vi "Process.vi"(8 "error in":errorcluster, 11 "Example Instrument UI":refnum<class "LevyLab Instrument UI.lvclass">) -> (0 "error out":errorcluster, 3 "Example Instrument UI out":refnum<class "LevyLab Instrument UI.lvclass">)   [LabVIEW 2016, in "LevyLab Instrument UI.lvclass"]
doc: "---------------------------------------------------------------\nJKI State Machine Objects™\nhttp://jki.net/state-machine-objects/\nCopyright (C) 2005-2015, JKI <info@jki.net>\nALL RIGHTS RESERVEDJKI State Machine Objects (SMO) 1.0.0.5\nJKI - JKI\nCopyright (c) 2016, JKI"
uses:
  LevyLab Instrument UI.lvclass
  C:/Program Files (x86)/National Instruments/LabVIEW 2016/vi.lib/JKI/JKI SMO/SMO/SMO.lvclass
  C:/Users/patrick/Documents/GitHub/Instrument-Framework/lvsrc/SMOs/Instrument UI/Instrument UI.lvclass
  C:/Program Files (x86)/National Instruments/LabVIEW 2016/vi.lib/JKI/JKI SMO/SMO.UI/SMO.UI.lvclass
  <vilib>/JKI/JKI SMO/SMO/Typedefs/Parent Call--Enum.ctl
  LevyLab Instrument/Typedefs/LevyLab Instrument.getAll--Cluster.ctl
  LevyLab Instrument/LevyLab Instrument.lvclass
  C:/Users/patrick/Documents/GitHub/Instrument-Framework/lvsrc/SMOs/Instrument/Instrument.lvclass
  SMOs/Instrument UI/Instrument UI.lvclass/Instrument UI.ctl
  SMOs/Instrument/Instrument.lvclass
  SMOs/Instrument UI/Instrument UI.lvclass
  <vilib>/JKI/JKI SMO/SMO/SMO.lvclass
  <vilib>/JKI/JKI SMO/SMO.UI/SMO.UI.lvclass
panel:
  out "Numeric":u32
  out "Instrument Response":dbl
  in  "Set Parameter":bool
  in  "Parameter":dbl
  in  "STOP":bool
  out "SMO string":string
  out "SMO Boolean":bool
  out "Logger SMO":dbl
  out "Levy 1":dbl
  # "#todo\nmake UI here. maybe include a nice picture of the hardware?"
  # "#todo\nadd buttons to do stuff (e.g., change a setting)\nButtons should trigger an event"
  # "#todo\nresize this box if you want your UI to be different size"
  # "SMO UI Template"
  # "For instructions on how to use the JKI State Machine Objects, examples and video tutorials, visit:\nhttp://jki.net/state-machine-objects/\n\nJKI State Machine Objects™\nhttp://jki.net/state-machine-objects/\nCopyright (C) 2005-2015, JKI <info@jki.net>\nALL RIGHTS RESERVED"
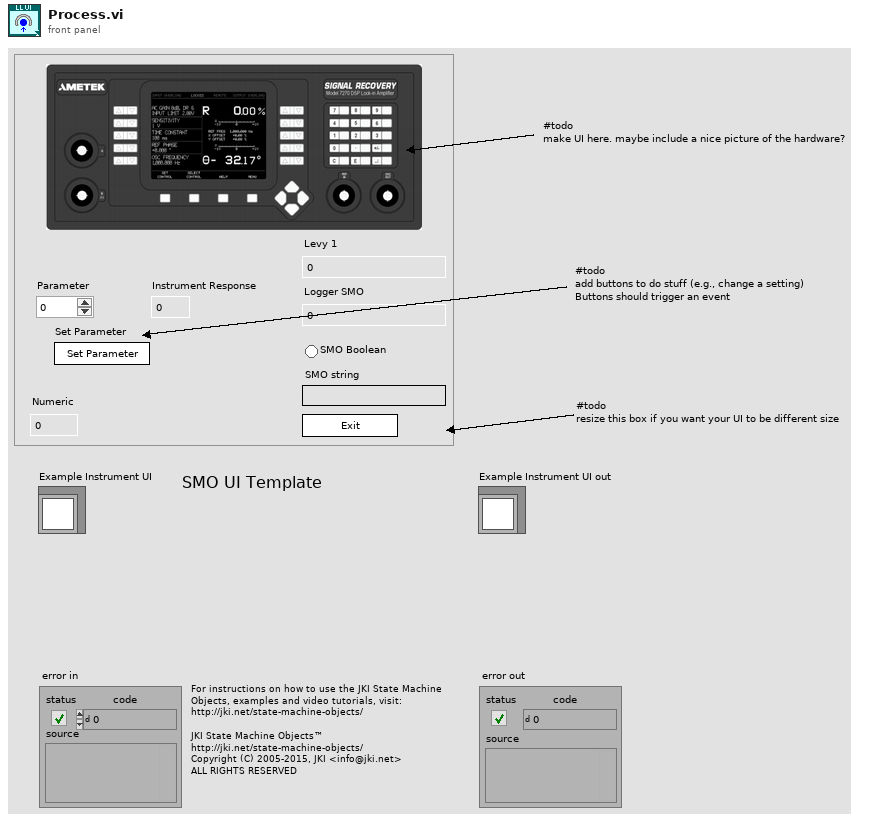
[diagram p1: front panel]
types:
  T1 = typedef "SMO.lvclass/Parent Call--Enum.ctl" = enum16{"Allows parent to run", "Does not request parent to run"}
  T2 = enum32{"invalid app kind", "Development System", "Run Time System", "Student Edition", "Embedded LabVIEW", "Evaluation", "Custom"}
  T3 = enum32{"Invalid", "Standard", "Closed", "Hidden", "Minimized", "Maximized"}
  T4 = typedef "LevyLab Instrument.lvclass/LevyLab Instrument.getAll--Cluster.ctl" = cluster{"Levy 1":dbl, "Logger SMO":dbl, "SMO Boolean":bool, "SMO String":string}
  T5 = cluster{"Core":cluster{"Current VI Reference":refnum<vi>, "Close Panel on Exit?":bool, "error":errorcluster}, "Instrument UI out":refnum<class "LevyLab Instrument UI.lvclass">, "Instrument":refnum<class "LevyLab Instrument.lvclass">, "getAll":T4, "Parameter":dbl}
  T6 = cluster{"Current VI Reference":refnum<vi>, "Close Panel on Exit?":bool, "error":errorcluster}
  T7 = typedef "SMO.lvclass/Protected Events.ctl" = cluster{"StopProcesses":refnum<user-event>, "AbortProcesses":refnum<user-event>, "Config Changed":refnum<user-event>, "Dependency":refnum<user-event>}
  T8 = typedef "Instrument.lvclass/PublicEvents--Cluster.ctl" = cluster{"MessageFromProcess":refnum<user-event>}
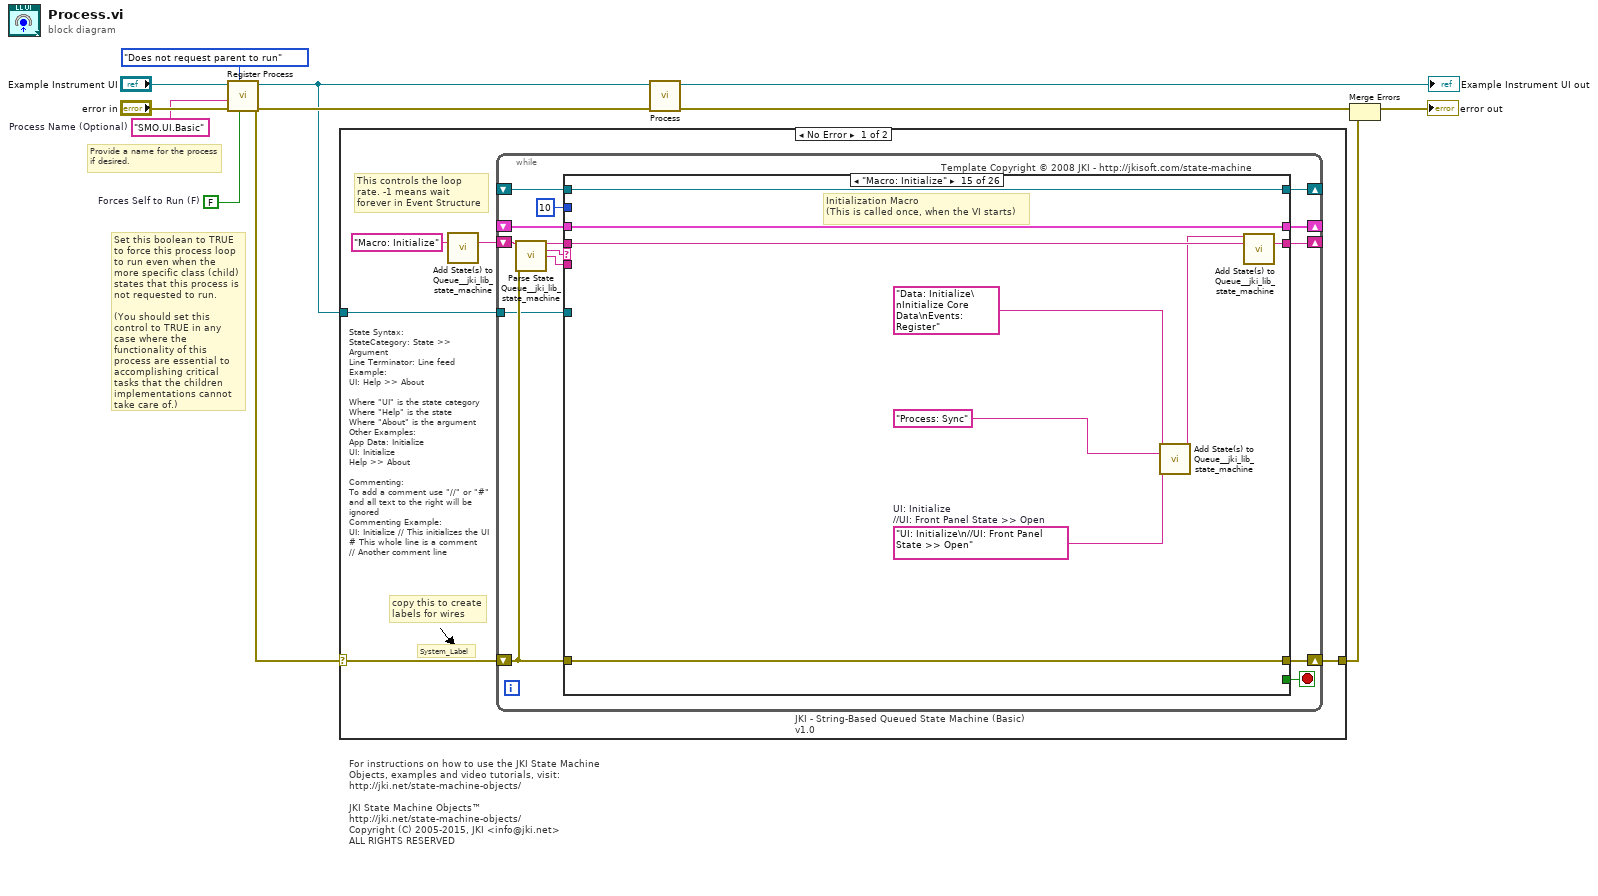
[diagram p0: block diagram]
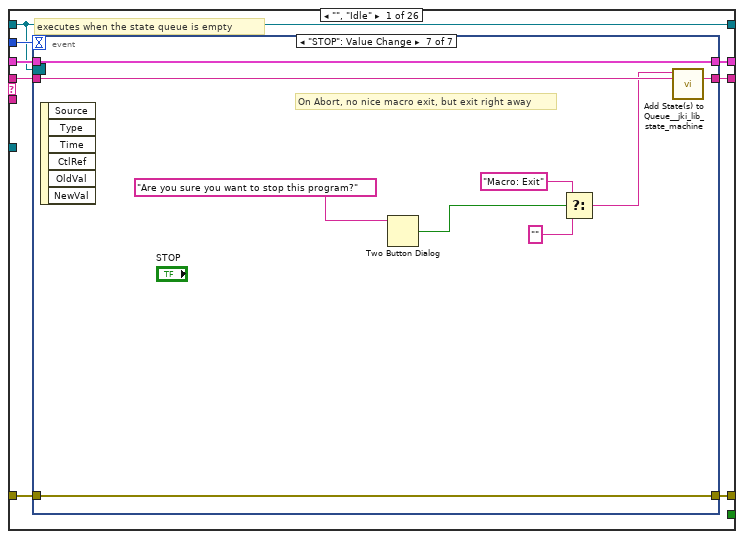
[diagram p2: hidden frame]
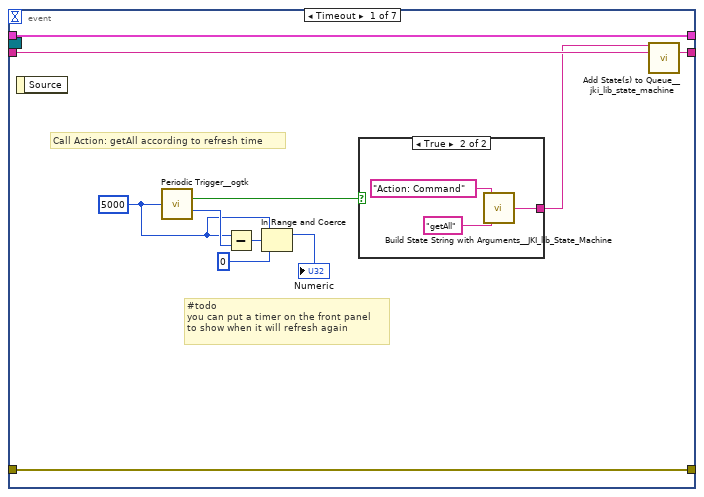
[diagram p3: hidden frame]
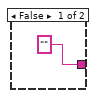
[diagram p4: hidden frame]
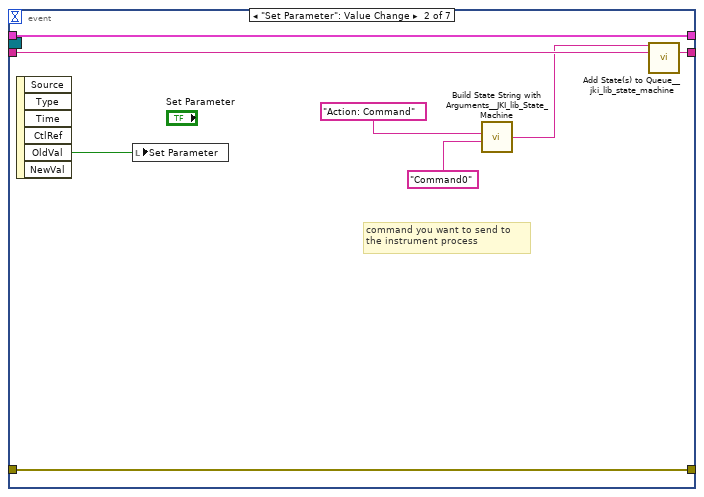
[diagram p5: hidden frame]
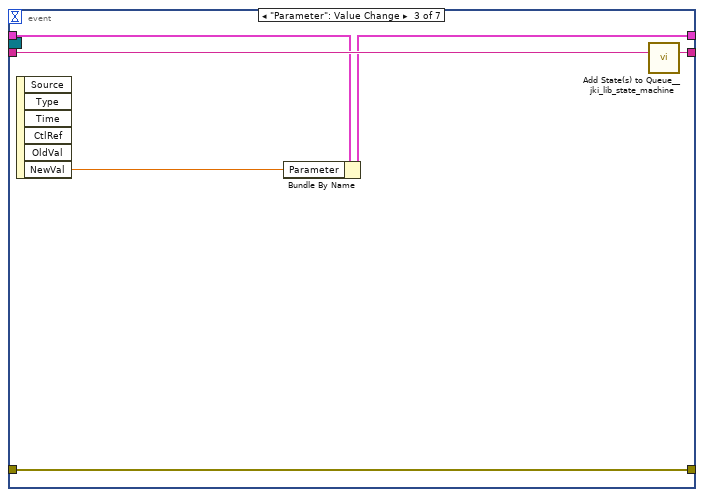
[diagram p6: hidden frame]
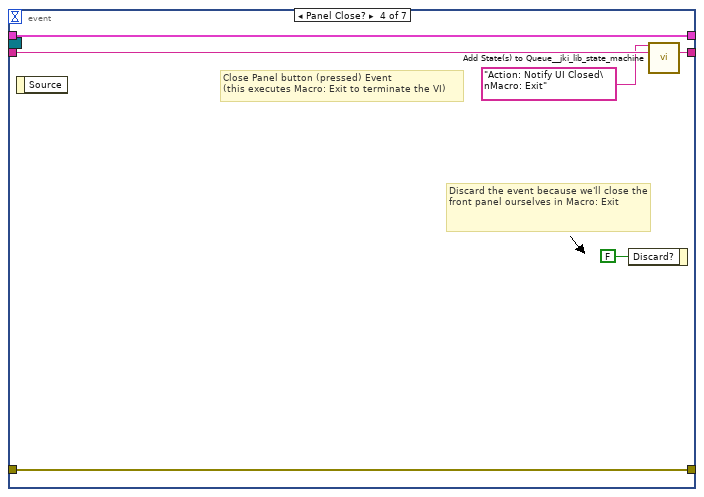
[diagram p7: hidden frame]
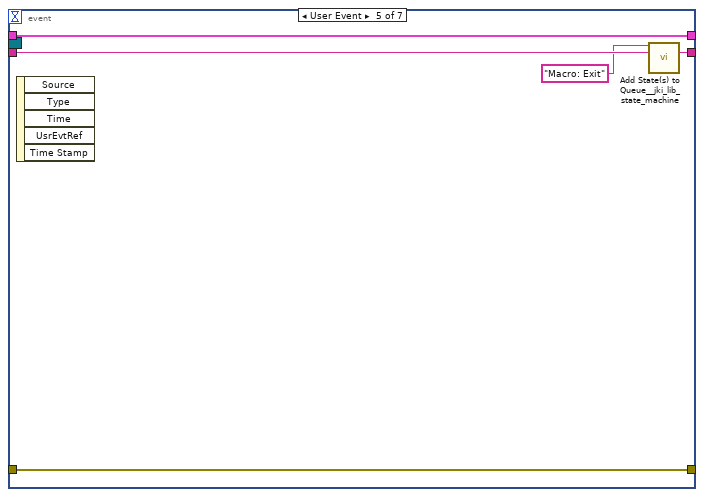
[diagram p8: hidden frame]
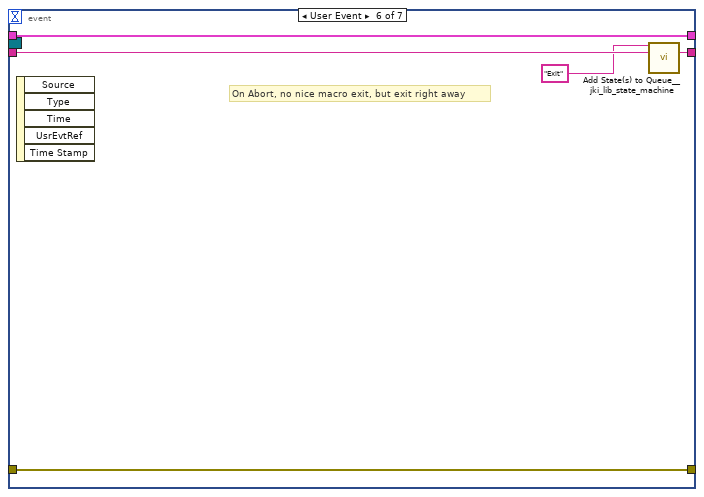
[diagram p9: hidden frame]
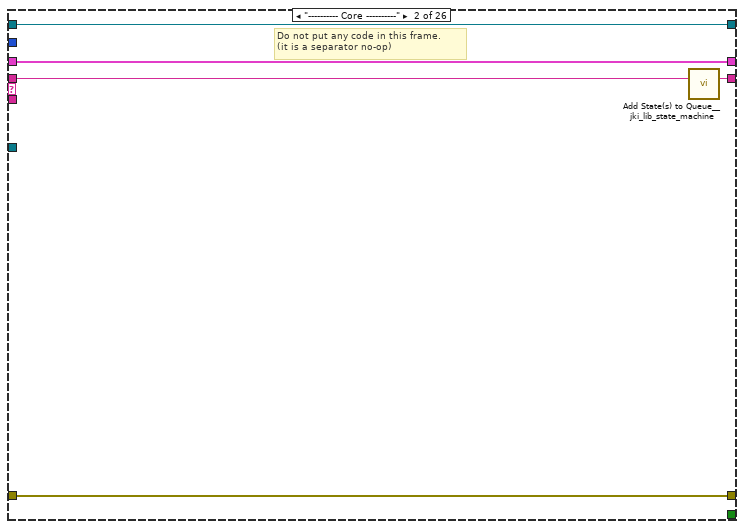
[diagram p10: hidden frame]
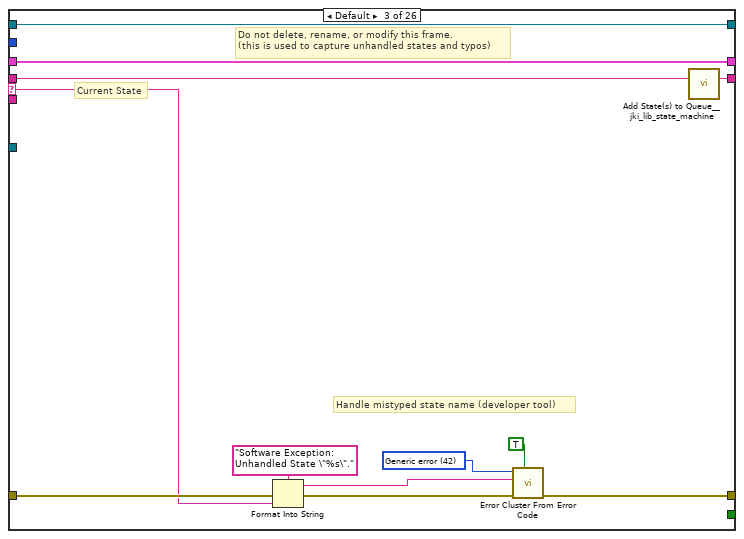
[diagram p11: hidden frame]
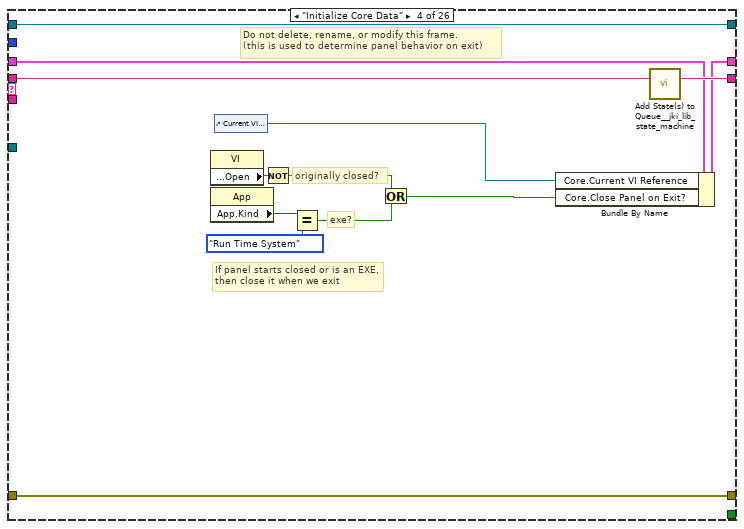
[diagram p12: hidden frame]
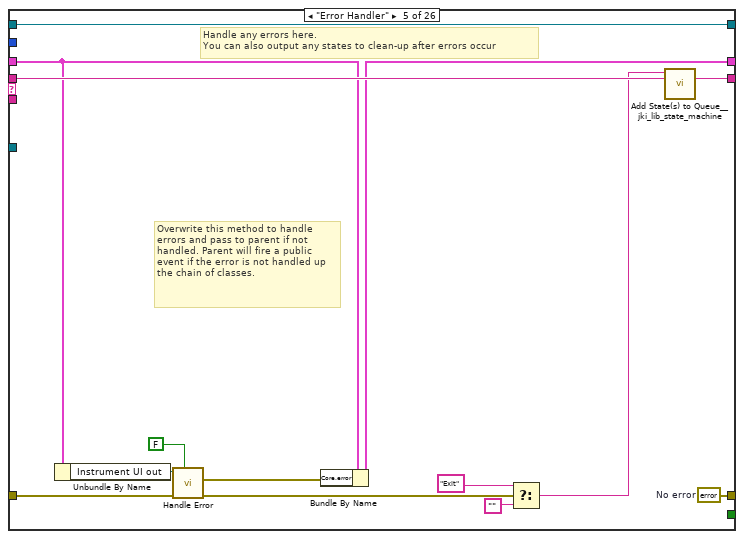
[diagram p13: hidden frame]
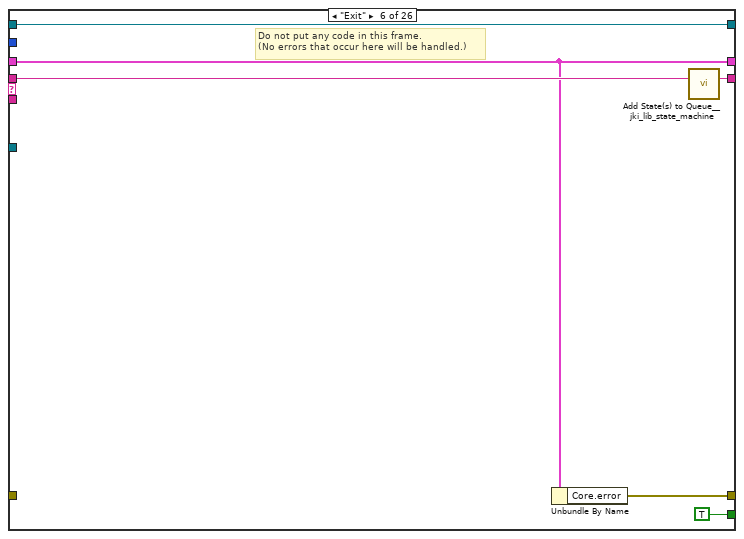
[diagram p14: hidden frame]
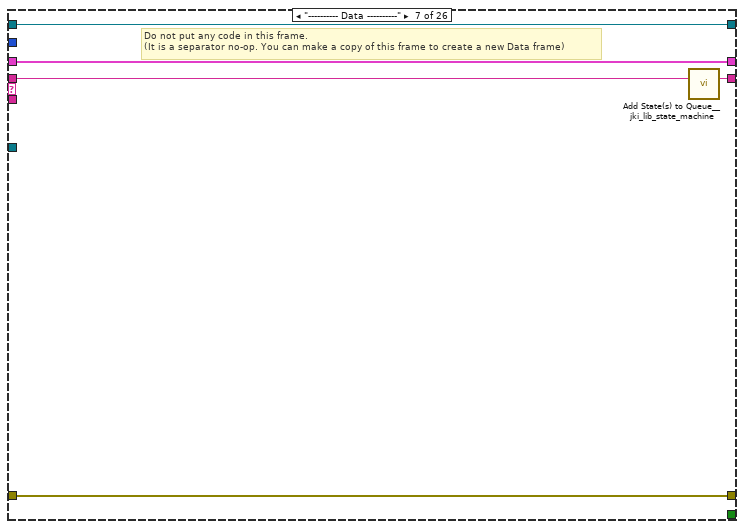
[diagram p15: hidden frame]
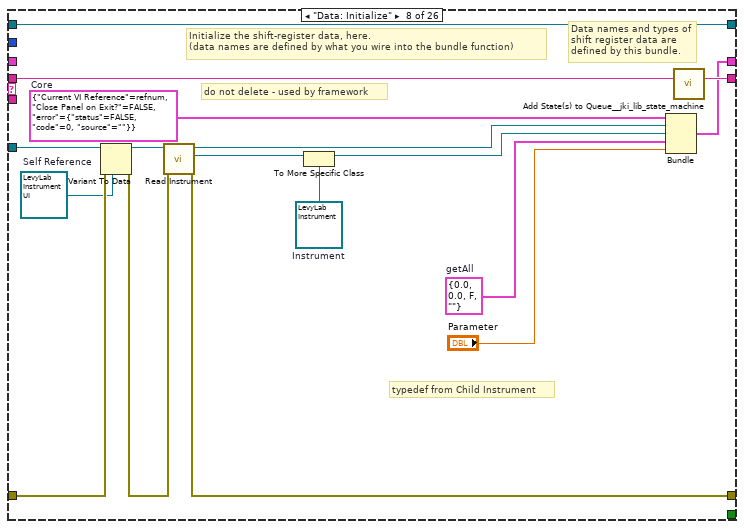
[diagram p16: hidden frame]
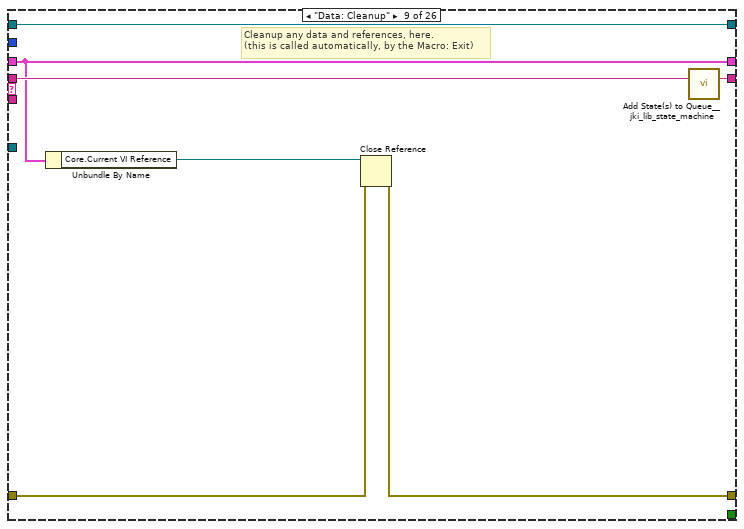
[diagram p17: hidden frame]
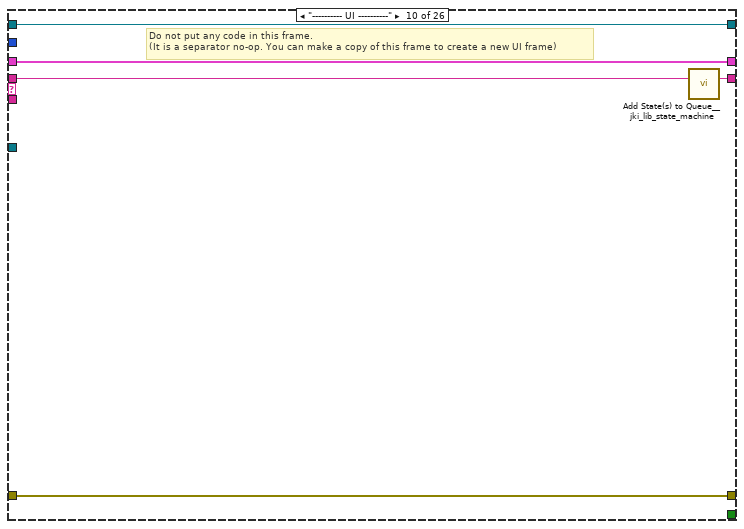
[diagram p18: hidden frame]
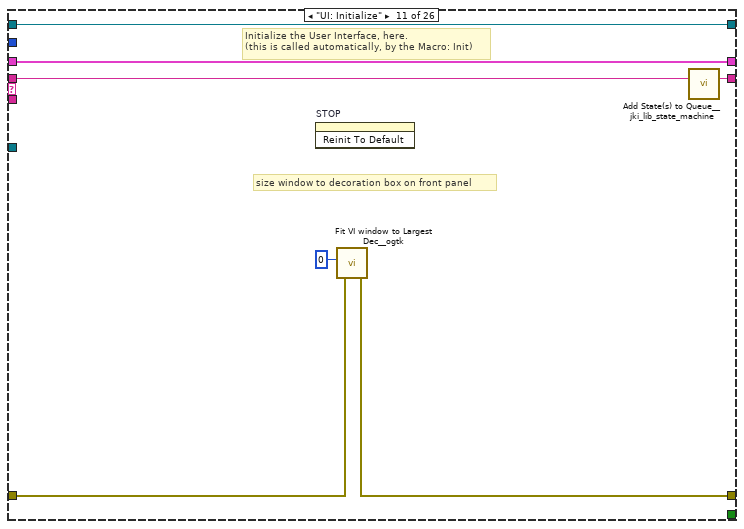
[diagram p19: hidden frame]
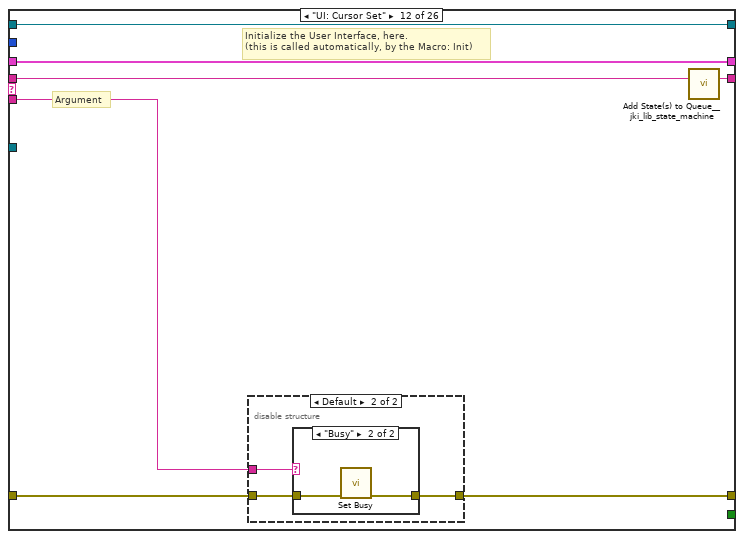
[diagram p20: hidden frame]
diagram:
  w2 = FALSE  # Forces Self to Run (F)
  w1 = "SMO.UI.Basic"  # Process Name (Optional)
  # "Provide a name for the process\nif desired."
  # "Set this boolean to TRUE to force this process loop to run even when the more specific class (child) states that this process is not requested to run.\n\n(You should set this control to TRUE in any case where the functionality of this process are essential to accomplishing critical tasks that the children implementations cannot take care of.)"
  # "For instructions on how to use the JKI State Machine Objects, examples and video tutorials, visit:\nhttp://jki.net/state-machine-objects/\n\nJKI State Machine Objects™\nhttp://jki.net/state-machine-objects/\nCopyright (C) 2005-2015, JKI <info@jki.net>\nALL RIGHTS RESERVED"
  n1 = call <vilib>:"Register Process.vi"("Forces Self to Run (F)"=w2, "Parent Call"=Parent_Call--Enum."Does not request parent to run", "error in (no error)"="error in", "Process Name (optional)"=w1, "SMO"="Example Instrument UI") -> ("error out"=w8:errorcluster, "SMO out"=w7:refnum<class "LevyLab Instrument UI.lvclass">)  [unwired: 5 in]
  n2 = case shown="No Error" w8 {
    selector: w8 -> [w13 w364]
    tunnel: w7 -> [w14 _]
    tunnel: [w12 w364] -> w4
    frame No Error {
      # "State Syntax:\nStateCategory: State >> Argument\nLine Terminator: Line feed\nExample:\nUI: Help >> About\n\nWhere \"UI\" is the state category\nWhere \"Help\" is the state\nWhere \"About\" is the argument\nOther Examples:\nApp Data: Initialize\nUI: Initialize\nHelp >> About\n\nCommenting:\nTo add a comment use \"//\" or \"#\" and all text to the right will be ignored\nCommenting Example:\nUI: Initialize // This initializes the UI\n# This whole line is a comment\n// Another comment line"
      # "copy this to create labels for wires"
      # "This controls the loop rate. -1 means wait forever in Event Structure"
      # "System_Label"
      n3 = call <vilib>:"Add State(s) to Queue__jki_lib_state_machine.vi"("State(s) in (\"\")"="Macro: Initialize") -> ("States Out"=w16:string)  [unwired: 14 in]
      n4 = while "JKI - String-Based Queued State Machine (Basic) v1.0" {
        shift-right: [w23] -> _
        shift-left: _ -> [w22]
        shift-right: [w26] -> w12
        shift-left: w13 -> [w20]
        shift-right: [w25] -> _
        shift-left: w16 -> [w27]
        tunnel: w14 -> [w19]
        shift-right: [w18] -> _
        shift-left: _ -> [w17]
        stop <- w24 stop-if-true
        # "Template Copyright © 2008 JKI - http://jkisoft.com/state-machine"
        n5 = call <vilib>:"Parse State Queue__jki_lib_state_machine.vi"("State Queue"=w27, "Error In (no error)"=w20) -> ("Remaining States"=w29:string, "Current State"=w30:string, "Arguments"=w28:string)  [unwired: 11 in]
        n6 = case shown="\"Macro: Initialize\"" w30 {
          selector: w30 -> [_ _ w99 _ _ _ _ _ _ _ _ _ _ _ _ _ _ _ _ _ _ _ _ _ _ _]
          tunnel: w29 -> [w38 w97 w103 w122 w136 w142 w147 w164 w171 w176 w183 w190 w206 w238 w247 w261 w266 w277 w284 w289 w302 w308 w315 w322 w332 w343]
          tunnel: w28 -> [_ _ _ _ _ _ _ _ _ _ _ w184 w200 _ _ _ _ _ _ _ _ _ _ _ _ w337]
          tunnel: w22 -> [w36 w94 w101 w113 w125 w138 w144 _ w166 w173 w181 w188 w202 w235 w243 w248 w263 w274 w279 w286 w300 w306 w311 w318 w329 w334]
          tunnel: [w35 w95 w105 w119 w127 w137 w145 w151 w167 w174 w178 w185 w203 w236 w245 w259 w264 w268 w280 w287 w295 w303 w312 w316 w323 w340] -> w26
          tunnel: w20 -> [w34 w95 w104 w119 w132 _ w145 w161 w168 w174 w179 w186 w204 w236 w245 w259 w264 w269 w281 w287 w297 w304 w312 w317 w323 w335]
          tunnel: [w37 w96 w102 w121 w135 w141 w146 w163 w170 w175 w182 w189 w205 w237 w246 w260 w265 w276 w283 w288 w301 w307 w314 w321 w331 w342] -> w25
          tunnel: [_ _ _ _ _ TRUE _ _ _ _ _ _ _ _ _ _ _ _ _ _ _ _ _ _ _ _] -> w24
          tunnel: [w33 w94 w101 w120 w124 w138 w144 w162 w166 w173 w181 w188 w202 w235 w243 w248 w263 w274 w279 w286 w300 w306 w310 w318 w329 w333] -> w23
          tunnel: 10 ("Timeout") -> [w32 _ _ _ _ _ _ _ _ _ _ _ _ _ _ _ _ _ _ _ _ _ _ _ _ _]
          tunnel: w19 -> [_ _ _ _ _ _ _ w159 _ _ _ _ _ _ _ _ _ _ _ _ _ _ _ _ _ _]
          tunnel: [w31 w93 w98 w110 w134 w139 w143 w158 w165 w172 w180 w187 w199 w234 w244 w253 w262 w275 w282 w285 w299 w305 w313 w320 w330 w341] -> w18
          tunnel: w17 -> [w31 w93 w98 w110 w134 w139 w143 w158 w165 w172 w180 w187 w199 w234 w244 w253 w262 w275 w282 w285 _ w305 w313 w320 w330 w341]
          frame "", "Idle" {
            # "executes when the state queue is empty"
            n7 = event shown="[6] \"STOP\": Value Change" {
              selector: w31 -> [_ _ _ _ _ _ _]
              dyn-events: _ -> [_ _ _ _ _ _ _]
              timeout: w32 -> [_ _ _ _ _ _ _]
              tunnel: w38 -> [w49 w61 w67 w73 w78 w83 w92]
              tunnel: [w48 w60 w66 w72 w77 w82 w91] -> w37
              tunnel: w36 -> [w46 w58 w63 w69 w75 w80 w89]
              tunnel: [w47 w59 w65 w68 w76 w81 w90] -> w35
              tunnel: w34 -> [w47 w59 w65 w68 w76 w81 w90]
              tunnel: [w46 w58 w62 w69 w75 w80 w89] -> w33
              event Timeout {
                w40 = u32 5000 ("time (ms)")
                # "#todo\nyou can put a timer on the front panel\nto show when it will refresh again"
                # "Call Action: getAll according to refresh time"
                n8 = event-data() -> ()  [unwired: 1 in, 1 out]
                n9 = call <userlib>:"Periodic Trigger__ogtk.vi"("time (ms)"=w40) -> ("Triggered"=w44:bool, "timer value"=w43:u32)  [unwired: 12 in, 1 out]
                n10 = Subtract(x=w40, y=w43) -> (x-y=w42:u32)
                n11 = In Range and Coerce(upper limit=w40, x=w42, lower limit=u32 0) -> (coerced(x)=→"Numeric":u32)  [unwired: 1 out]
                n12 = case shown="True" w44 {
                  tunnel: ["" ("State(s) in Front (\"\")") w51] -> w45
                  frame False {
                  }
                  frame True {
                    n13 = call <vilib>:"Build State String with Arguments__JKI_lib_State_Machine.vi"("Arguments (\"\")"="getAll" ("State(s) in Front (\"\")"), "State"="Action: Command" ("State(s) in Front (\"\")")) -> ("State with Arguments"=w51:string)  [unwired: 4 in]
                  }
                }
                n14 = call <vilib>:"Add State(s) to Queue__jki_lib_state_machine.vi"("State(s) in Front (\"\")"=w45, "State(s) in (\"\")"=w49) -> ("States Out"=w48:string)  [unwired: 13 in]
              }
              event "Set Parameter": Value Change {
                # "command you want to send to\nthe instrument process"
                n15 = event-data() -> ("OldVal"=w57:bool)  [unwired: 1 in, 5 out]
                n16 = local write "Set Parameter"(w57) -> ()
                n17 = call <vilib>:"Build State String with Arguments__JKI_lib_State_Machine.vi"("Arguments (\"\")"="Command0" ("State(s) in Front (\"\")"), "State"="Action: Command" ("State(s) in Front (\"\")")) -> ("State with Arguments"=w54:string)  [unwired: 4 in]
                n18 = call <vilib>:"Add State(s) to Queue__jki_lib_state_machine.vi"("State(s) in Front (\"\")"=w54, "State(s) in (\"\")"=w61) -> ("States Out"=w60:string)  [unwired: 13 in]
              }
              event "Parameter": Value Change {
                n19 = event-data() -> ("NewVal"=w64:dbl)  [unwired: 1 in, 5 out]
                n20 = Bundle By Name(cluster=w63, "Parameter"=w64) -> (w62:T5)
                n21 = call <vilib>:"Add State(s) to Queue__jki_lib_state_machine.vi"("State(s) in (\"\")"=w67) -> ("States Out"=w66:string)  [unwired: 14 in]
              }
              event Panel Close? {
                # "Discard the event because we'll close the front panel ourselves in Macro: Exit"
                # "Close Panel button (pressed) Event\n(this executes Macro: Exit to terminate the VI)"
                n22 = event-data() -> ()  [unwired: 1 in, 1 out]
                n23 = event-data("Discard?"=FALSE) -> ()  [unwired: 1 in, 1 out]
                n24 = call <vilib>:"Add State(s) to Queue__jki_lib_state_machine.vi"("State(s) in Front (\"\")"="Action: Notify UI Closed\nMacro: Exit", "State(s) in (\"\")"=w73) -> ("States Out"=w72:string)  [unwired: 13 in]
              }
              event User Event {
                n25 = event-data() -> ()  [unwired: 1 in, 5 out]
                n26 = call <vilib>:"Add State(s) to Queue__jki_lib_state_machine.vi"("State(s) in Front (\"\")"="Macro: Exit", "State(s) in (\"\")"=w78) -> ("States Out"=w77:string)  [unwired: 13 in]
              }
              event User Event {
                # "On Abort, no nice macro exit, but exit right away"
                n27 = event-data() -> ()  [unwired: 1 in, 5 out]
                n28 = call <vilib>:"Add State(s) to Queue__jki_lib_state_machine.vi"("State(s) in Front (\"\")"="Exit", "State(s) in (\"\")"=w83) -> ("States Out"=w82:string)  [unwired: 13 in]
              }
              event "STOP": Value Change {
                # "On Abort, no nice macro exit, but exit right away"
                n29 = event-data() -> ()  [unwired: 1 in, 6 out]
                n30 = Two Button Dialog(message="Are you sure you want to stop this program?") -> (T button?=w88:bool)  [unwired: 2 in]
                n31 = Select(t="Macro: Exit", s=w88, f="") -> (s? t:f=w84:string)
                n32 = call <vilib>:"Add State(s) to Queue__jki_lib_state_machine.vi"("State(s) in Front (\"\")"=w84, "State(s) in (\"\")"=w92) -> ("States Out"=w91:string)  [unwired: 13 in]
              }
            }
          }
          frame "---------- Core ----------" {
            # "Do not put any code in this frame.\n(it is a separator no-op)"
            n33 = call <vilib>:"Add State(s) to Queue__jki_lib_state_machine.vi"("State(s) in (\"\")"=w97) -> ("States Out"=w96:string)  [unwired: 14 in]
          }
          frame Default {
            w108 = 42 items=["No error", "Argument error", "Memory is full", "Out of zone", "End of file", "File already open", "Generic file I/O error", "File not found", "File permission error", "Disk is full", "Duplicate path", "Too many files open", "System feature not enabled", "Resource file not found", "Cannot add resource", "Resource not found", "Image not found", "Image memory error", "Pen does not exist", "Config type invalid", "Config token not found", "Config parse error", "Config memory error", "Bad external code format", "Bad external code offset", "External code not present", "Null window", "Destroy window error", "Null menu", "Print aborted", "Bad print record", "Print driver error", "Windows error during printing", "Memory error during printing", "Print dialog error", "Generic print error", "Invalid device refnum", "Device not found", "Device parameter error", "Device unit error", "Cannot open device", "Device call aborted", "Generic error", "Cancelled by user", "Object ID too low", "Object ID too high", "Object not in heap", "Unknown heap", "Unknown object (invalid DefProc)", "Unknown object (DefProc not in table)", "Message out of range", "Invalid (null) method", "Unknown message", "Manager call not supported", "Bad address", "Network operation in progress", "Network operation timed out", "Connection is busy", "Network attribute not supported", "Network error", "Address in use", "System out of memory", "Connection aborted", "Connection refused", "Not connected", "Already connected", "Connection closed", "Initialization error (interapplication manager)", "Bad occurrence", "Wait on unbound occurrence handler", "Occurrence queue overflow", "Datalog type conflict", "Unused", "Unrecognized type (interapplication manager)", "Memory corrupt", "Failed to make temporary DLL", "Old CIN version", "Drag socket not found", "Failed to load drop-object", "Failed to register OLE object", "Failed to release OLE object", "Format specifier type mismatch", "Unknown format specifier", "Too few format specifiers", "Too many format specifiers", "Scan failed", "Newer CIN version", "Error converting to variant", "Runtime menu error", "Password tampered", "Variant attribute not found", "Incompatible variant data type", "Event data is not available", "Event Store is not present", "Occurrence is not found", "Event Queue is not created", "Event info is not available", "Refnum passed is NULL", "Error retrieving Class GUID", "Error retrieving CoClass GUID", "Error retrieving TypeLib GUID.", "Bad built application magic bytes.", "Specific driver is different from the specific driver associated with the Logical Name.", "There is no session opened to the class driver.", "Max Error", "MAX - Error with config objects", "MAX - Error loading configuration", "MAX - Group not supported"]
            # "Current State"
            # "Do not delete, rename, or modify this frame.\n(this is used to capture unhandled states and typos)"
            # "Handle mistyped state name (developer tool)"
            n34 = Format Into String(format string="Software Exception: Unhandled State \"%s\"." ("message"), error in=w104, w99) -> (resulting string=w107:string, error out=w106:errorcluster)  [unwired: 1 in]
            n35 = call <vilib>:"Error Cluster From Error Code.vi"("show call chain? (False)"=TRUE, "error in (no error)"=w106, "error message (\"\")"=w107, "error code (0)"=w108) -> ("error out"=w105:errorcluster)  [unwired: 5 in]
            n36 = call <vilib>:"Add State(s) to Queue__jki_lib_state_machine.vi"("State(s) in (\"\")"=w103) -> ("States Out"=w102:string)  [unwired: 14 in]
          }
          frame "Initialize Core Data" {
            # "Do not delete, rename, or modify this frame.\n(this is used to determine panel behavior on exit)"
            # "originally closed?"
            # "exe?"
            # "If panel starts closed or is an EXE, then close it when we exit"
            n37 = property class="VI"() -> ("Front Panel.Open"=w118:bool)  [unwired: 2 in, 2 out]
            n38 = property class="App"() -> ("App.Kind"=w117:T2)  [unwired: 2 in, 2 out]
            n39 = control-ref of="Current VI Reference"() -> (w111:refnum<vi>)
            n40 = Not(x=w118) -> (.not. x?=w115:bool)
            n41 = Equal?(x=w117, y=T2."Run Time System" ("Application:Kind")) -> (x = y?=w114:bool)
            n42 = Or(x=w115, y=w114) -> (x .or. y?=w112:bool)
            n43 = Bundle By Name(cluster=w113, "Core.Current VI Reference"=w111, "Core.Close Panel on Exit?"=w112) -> (w120:T5)
            n44 = call <vilib>:"Add State(s) to Queue__jki_lib_state_machine.vi"("State(s) in (\"\")"=w122) -> ("States Out"=w121:string)  [unwired: 14 in]
          }
          frame "Error Handler" {
            w127 = errorcluster {"status"=FALSE, "code"=0, "source"=""}  # No error
            # "Overwrite this method to handle errors and pass to parent if not handled. Parent will fire a public event if the error is not handled up the chain of classes."
            # "Handle any errors here.\nYou can also output any states to clean-up after errors occur"
            n45 = Unbundle By Name(w125) -> ("Instrument UI out"=w133:refnum<class "LevyLab Instrument UI.lvclass">)
            n46 = call-dynamic "Handle Error.vi"("Stop on Unhandled Error (T)"=FALSE, "error in"=w132, "Instrument UI"=w133) -> ("handling error"=w128:errorcluster, "Unhandled error"=w126:errorcluster)  [unwired: 6 in, 1 out]
            n47 = Bundle By Name(cluster=w125, "Core.error"=w126) -> (w124:T5)
            n48 = Select(t="Exit", s=w128, f="") -> (s? t:f=w129:string)
            n49 = call <vilib>:"Add State(s) to Queue__jki_lib_state_machine.vi"("State(s) in Front (\"\")"=w129, "State(s) in (\"\")"=w136) -> ("States Out"=w135:string)  [unwired: 13 in]
          }
          frame "Exit" {
            # "Do not put any code in this frame.\n(No errors that occur here will be handled.)"
            n50 = Unbundle By Name(w138) -> ("Core.error"=w137:errorcluster)
            n51 = call <vilib>:"Add State(s) to Queue__jki_lib_state_machine.vi"("State(s) in (\"\")"=w142) -> ("States Out"=w141:string)  [unwired: 14 in]
          }
          frame "---------- Data ----------" {
            # "Do not put any code in this frame.\n(It is a separator no-op. You can make a copy of this frame to create a new Data frame)"
            n52 = call <vilib>:"Add State(s) to Queue__jki_lib_state_machine.vi"("State(s) in (\"\")"=w147) -> ("States Out"=w146:string)  [unwired: 14 in]
          }
          frame "Data: Initialize" {
            w154 = refnum<class "LevyLab Instrument.lvclass"> refnum  # Instrument
            w155 = T4 {"Levy 1"=0.0, "Logger SMO"=0.0, "SMO Boolean"=FALSE, "SMO String"=""}  # getAll
            w157 = T6 {"Current VI Reference"=refnum, "Close Panel on Exit?"=FALSE, "error"={"status"=FALSE, "code"=0, "source"=""}}  # Core
            w160 = refnum<class "LevyLab Instrument UI.lvclass"> refnum  # Self Reference
            # "typedef from Child Instrument"
            # "do not delete - used by framework"
            # "Data names and types of shift register data are defined by this bundle."
            # "Initialize the shift-register data, here.\n(data names are defined by what you wire into the bundle function)"
            n53 = Variant To Data(error in=w161, type=w160, Variant=w159) -> (data=w149:refnum<class "LevyLab Instrument UI.lvclass">, error out=w152:errorcluster)
            n54 = call "Read Instrument.vi"("error in (no error)"=w152, "Instrument UI in"=w149) -> ("error out"=w151:errorcluster, "Instrument.lvclass"=w150:refnum<class "Instrument.lvclass">, "Instrument UI out"=w148:refnum<class "LevyLab Instrument UI.lvclass">)  [unwired: 7 in]
            n55 = To More Specific Class(target class=w154, reference=w150) -> (specific class reference=w153:refnum<class "LevyLab Instrument.lvclass">)  [unwired: 1 in, 1 out]
            n56 = Bundle("Core"=w157, "Instrument UI out"=w148, "Instrument"=w153, "getAll"=w155, "Parameter"="Parameter") -> (w162:T5)  [unwired: 1 in]
            n57 = call <vilib>:"Add State(s) to Queue__jki_lib_state_machine.vi"("State(s) in (\"\")"=w164) -> ("States Out"=w163:string)  [unwired: 14 in]
          }
          frame "Data: Cleanup" {
            # "Cleanup any data and references, here.\n(this is called automatically, by the Macro: Exit)"
            n58 = Unbundle By Name(w166) -> ("Core.Current VI Reference"=w169:refnum<vi>)
            n59 = Close Reference(reference=w169, error in (no error)=w168) -> (error out=w167:errorcluster)
            n60 = call <vilib>:"Add State(s) to Queue__jki_lib_state_machine.vi"("State(s) in (\"\")"=w171) -> ("States Out"=w170:string)  [unwired: 14 in]
          }
          frame "---------- UI ----------" {
            # "Do not put any code in this frame.\n(It is a separator no-op. You can make a copy of this frame to create a new UI frame)"
            n61 = call <vilib>:"Add State(s) to Queue__jki_lib_state_machine.vi"("State(s) in (\"\")"=w176) -> ("States Out"=w175:string)  [unwired: 14 in]
          }
          frame "UI: Initialize" {
            # "size window to decoration box on front panel"
            # "Initialize the User Interface, here.\n(this is called automatically, by the Macro: Init)"
            n62 = invoke on="STOP" class="Bool (strict)" method="Reinit To Default"() -> ()  [unwired: 3 in, 3 out]
            n63 = call <userlib>:"Fit VI window to Largest Dec__ogtk.vi"("error in (no error)"=w179, "border spacing (2 px)"=0) -> ("error out"=w178:errorcluster)  [unwired: 4 in, 1 out]
            n64 = call <vilib>:"Add State(s) to Queue__jki_lib_state_machine.vi"("State(s) in (\"\")"=w183) -> ("States Out"=w182:string)  [unwired: 14 in]
          }
          frame "UI: Cursor Set" {
            # "Argument"
            # "Initialize the User Interface, here.\n(this is called automatically, by the Macro: Init)"
            n65 = disable-structure shown="Default" {
              disable-tunnel: w186 -> [w191 w194]
              disable-tunnel: [w191 w193] -> w185
              disable-tunnel: w184 -> [_ w192]
              frame condition #0 {
              }
              frame condition #1 (active) {
                n66 = case shown="\"Busy\"" w192 {
                  tunnel: w194 -> [w196 w198]
                  tunnel: [w195 w197] -> w193
                  frame "Idle", Default {
                    n67 = call <vilib>:"Unset Busy.vi"("error in (no error)"=w196) -> ("error out"=w195:errorcluster)  [unwired: 10 in]
                  }
                  frame "Busy" {
                    n68 = call <vilib>:"Set Busy.vi"("error in (no error)"=w198) -> ("error out"=w197:errorcluster)  [unwired: 9 in, 1 out]
                  }
                }
              }
            }
            n69 = call <vilib>:"Add State(s) to Queue__jki_lib_state_machine.vi"("State(s) in (\"\")"=w190) -> ("States Out"=w189:string)  [unwired: 14 in]
          }
          frame "UI: Front Panel State" {
            # "Argument"
            # "Set Front Panel Open or Closed\n(Usage: \"UI: Front Panel State >> Open|Close\")"
            n70 = Unbundle By Name(w202) -> ("Core.Current VI Reference"=w201:refnum<vi>)
            n71 = disable-structure shown="Default" {
              disable-tunnel: w204 -> [w210 w233]
              disable-tunnel: [w209 w233] -> w203
              disable-tunnel: w201 -> [w208 _]
              disable-tunnel: w200 -> [w207 _]
              frame condition #0 (active) {
                n72 = case shown="\"Close\"" w207 {
                  tunnel: w210 -> [w214 w227]
                  tunnel: [w216 w228] -> w209
                  tunnel: w208 -> [w215 w225]
                  frame "Open", Default {
                    n73 = property class="VI"(reference=w215, error in=w214) -> (reference out=w212:refnum<vi>, error out=w213:errorcluster, "FP.State"=w211:T3)
                    n74 = case shown="\"Closed\"" w211 {
                      tunnel: [w219 w222] -> w216
                      tunnel: w213 -> [w218 w222]
                      tunnel: w212 -> [w217 _]
                      frame "Closed" {
                        n75 = invoke class="VI" method="FP.Open"(reference=w217, error in=w218, "Activate"=TRUE, "State"=T3."Standard") -> (error out=w219:errorcluster)  [unwired: 1 in, 4 out]
                      }
                      frame Default {
                      }
                    }
                  }
                  frame "Close" {
                    n76 = property class="VI"(reference=w225, error in=w227) -> (reference out=w224:refnum<vi>, error out=w226:errorcluster, "FP.State"=w223:T3)
                    n77 = case shown="Default" w223 {
                      tunnel: [w229 w232] -> w228
                      tunnel: w226 -> [w229 w231]
                      tunnel: w224 -> [_ w230]
                      frame "Invalid", "Closed" {
                      }
                      frame Default {
                        n78 = invoke class="VI" method="FP.Close"(reference=w230, error in=w231) -> (error out=w232:errorcluster)  [unwired: 1 in, 2 out]
                      }
                    }
                  }
                }
              }
              frame condition #1 {
              }
            }
            n79 = call <vilib>:"Add State(s) to Queue__jki_lib_state_machine.vi"("State(s) in (\"\")"=w206) -> ("States Out"=w205:string)  [unwired: 14 in]
          }
          frame "---------- Macro ----------" {
            # "Do not put any code in this frame.\n(It is a separator no-op. You can make a copy of this frame to create a new Macro frame)"
            n80 = call <vilib>:"Add State(s) to Queue__jki_lib_state_machine.vi"("State(s) in (\"\")"=w238) -> ("States Out"=w237:string)  [unwired: 14 in]
          }
          frame "Macro: Initialize" {
            w241 = "UI: Initialize\n//UI: Front Panel State >> Open"  # UI: Initialize //UI: Front Panel State >> Open
            # "Initialization Macro\n(This is called once, when the VI starts)"
            n81 = call <vilib>:"Add State(s) to Queue__jki_lib_state_machine.vi"("State(s) in Front (\"\")"="Data: Initialize\nInitialize Core Data\nEvents: Register", "State(s) in (\"\")"="Process: Sync", "State(s) at Back (\"\")"=w241) -> ("States Out"=w240:string)  [unwired: 12 in]
            n82 = call <vilib>:"Add State(s) to Queue__jki_lib_state_machine.vi"("State(s) in Front (\"\")"=w240, "State(s) in (\"\")"=w247) -> ("States Out"=w246:string)  [unwired: 13 in]
          }
          frame "Macro: Exit" {
            # "Exit Macro\n(This is called once, when the VI exits)"
            n83 = Unbundle By Name(w248) -> ("Core.Close Panel on Exit?"=w258:bool)
            n84 = Select(t="UI: Front Panel State >> Close", s=w258, f="") -> (s? t:f=w255:string)
            n85 = call <vilib>:"Add State(s) to Queue__jki_lib_state_machine.vi"("State(s) in Front (\"\")"="Data: Cleanup\nEvents: Unregister\nProcess: Self Terminate", "State(s) in (\"\")"="Process: Sync", "State(s) at Back (\"\")"="Exit") -> ("States Out"=w250:string)  [unwired: 12 in]
            n86 = call <vilib>:"Add State(s) to Queue__jki_lib_state_machine.vi"("State(s) in (\"\")"=w255, "State(s) at Back (\"\")"=w250) -> ("States Out"=w254:string)  [unwired: 13 in]
            n87 = call <vilib>:"Add State(s) to Queue__jki_lib_state_machine.vi"("State(s) in Front (\"\")"=w254, "State(s) in (\"\")"=w261) -> ("States Out"=w260:string)  [unwired: 13 in]
          }
          frame "---------- Process ----------" {
            # "Template Separator\n(You can make a copy of, or modify, this frame)"
            n88 = call <vilib>:"Add State(s) to Queue__jki_lib_state_machine.vi"("State(s) in (\"\")"=w266) -> ("States Out"=w265:string)  [unwired: 14 in]
          }
          frame "Process: Sync" {
            n89 = Unbundle By Name(w274) -> ("Instrument UI out"=w270:refnum<class "LevyLab Instrument UI.lvclass">)
            n90 = call <vilib>:"WaitOnProcessSync.vi"("error in (no error)"=w269, "SMO"=w270) -> ("error out"=w268:errorcluster, "Don't run?"=w273:bool)  [unwired: 7 in, 1 out]
            n91 = Select(t="Data: Cleanup\nEvents: Unregister\nExit", s=w273, f="") -> (s? t:f=w267:string)
            n92 = call <vilib>:"Add State(s) to Queue__jki_lib_state_machine.vi"("State(s) in Front (\"\")"=w267, "State(s) in (\"\")"=w277) -> ("States Out"=w276:string)  [unwired: 13 in]
          }
          frame "Process: Self Terminate" {
            n93 = Unbundle By Name(w279) -> ("Instrument UI out"=w278:refnum<class "LevyLab Instrument UI.lvclass">)
            n94 = call <vilib>:"SelfTerminate.vi"("error in (no error)"=w281, "SMO in"=w278) -> ("error out"=w280:errorcluster)  [unwired: 8 in, 1 out]
            n95 = call <vilib>:"Add State(s) to Queue__jki_lib_state_machine.vi"("State(s) in (\"\")"=w284) -> ("States Out"=w283:string)  [unwired: 14 in]
          }
          frame "---------- Events ----------" {
            # "Template Separator\n(You can make a copy of, or modify, this frame)"
            n96 = call <vilib>:"Add State(s) to Queue__jki_lib_state_machine.vi"("State(s) in (\"\")"=w289) -> ("States Out"=w288:string)  [unwired: 14 in]
          }
          frame "Events: Register" {
            # "Expand to add\nmore events"
            # "Base Class Protected Events"
            n97 = Unbundle By Name(w300) -> ("Instrument UI out"=w290:refnum<class "LevyLab Instrument UI.lvclass">, "Instrument"=w293:refnum<class "LevyLab Instrument.lvclass">)
            n98 = call <vilib>:"GetProtectedEvents.vi"("SMO"=w290) -> ("error out"=w294:errorcluster, "SMO Protected Events"=w298:T7)  [unwired: 8 in, 1 out]
            n99 = call "Instrument.GetPublicEvents.vi"("Instrument"=w293) -> ("error out"=w291:errorcluster, "Instrument Public Events"=w292:T8)  [unwired: 8 in, 1 out]
            n100 = register-events(w298, w292) -> (reference out=w299:refnum<event-registration>, error out=w296:errorcluster)  [unwired: 2 in]
            n101 = Merge Errors(w291, w297, w296, w294) -> (w295:errorcluster)
            n102 = call <vilib>:"Add State(s) to Queue__jki_lib_state_machine.vi"("State(s) in (\"\")"=w302) -> ("States Out"=w301:string)  [unwired: 14 in]
          }
          frame "Events: Unregister" {
            n103 = Unregister For Events(event registration refnum=w305, error in=w304) -> (error out=w303:errorcluster)
            n104 = call <vilib>:"Add State(s) to Queue__jki_lib_state_machine.vi"("State(s) in (\"\")"=w308) -> ("States Out"=w307:string)  [unwired: 14 in]
          }
          frame "---------- Action ----------" {
            n105 = Unbundle By Name(w311) -> ("Instrument UI out"=w309:refnum<class "LevyLab Instrument UI.lvclass">)
            n106 = Bundle By Name(cluster=w311, "Instrument UI out"=w309) -> (w310:T5)
            n107 = call <vilib>:"Add State(s) to Queue__jki_lib_state_machine.vi"("State(s) in (\"\")"=w315) -> ("States Out"=w314:string)  [unwired: 14 in]
          }
          frame "Action: Notify UI Closed" {
            # "Notify that the UI has been closed"
            n108 = Unbundle By Name(w318) -> ("Instrument UI out"=w319:refnum<class "LevyLab Instrument UI.lvclass">)
            n109 = call <vilib>:"Hide.vi"("error in (no error)"=w317, "SMO.UI"=w319) -> ("error out"=w316:errorcluster)  [unwired: 8 in, 1 out]
            n110 = call <vilib>:"Add State(s) to Queue__jki_lib_state_machine.vi"("State(s) in (\"\")"=w322) -> ("States Out"=w321:string)  [unwired: 14 in]
          }
          frame "Action: Update Front Panel" {
            # "do this way to have nicer UI or only display what you want"
            n111 = Unbundle By Name(w329) -> ("getAll"=w324:T4)
            n112 = Unbundle By Name(w324) -> ("Levy 1"=→"Levy 1":dbl, "Logger SMO"=→"Logger SMO":dbl, "SMO Boolean"=→"SMO Boolean":bool, "SMO String"=→"SMO string":string)
            n113 = call <vilib>:"Add State(s) to Queue__jki_lib_state_machine.vi"("State(s) in (\"\")"=w332) -> ("States Out"=w331:string)  [unwired: 14 in]
          }
          frame "Action: Command" {
            # "command"
            n114 = Unbundle By Name(w334) -> ("Instrument"=w338:refnum<class "LevyLab Instrument.lvclass">, "Parameter"=w336:dbl)
            n115 = case shown="\"getAll\"" w337 {
              tunnel: w336 -> [_ _ w363]
              tunnel: w335 -> [w346 w353 w361]
              tunnel: [w346 w351 w357] -> w340
              tunnel: ["" ("State(s) in Front (\"\")") "Action: Update Front Panel" ("State(s) in Front (\"\")") "" ("State(s) in Front (\"\")")] -> w339
              tunnel: w338 -> [_ w354 _]
              tunnel: w334 -> [w344 w350 w358]
              tunnel: [w344 w355 w358] -> w333
              frame Default {
              }
              frame "getAll" {
                n116 = Unbundle By Name(w350) -> ("getAll"=w349:T4)
                n117 = call "GET ALL.vi"("error in (no error)"=w353, "Instrument in"=w354) -> ("error out"=w352:errorcluster, "getAll"=w347:variant)  [unwired: 7 in, 1 out]
                n118 = Variant To Data(error in=w352, type=w349, Variant=w347) -> (data=w348:T4, error out=w351:errorcluster)
                n119 = Bundle By Name(cluster=w350, "getAll"=w348) -> (w355:T5)
              }
              frame "Command0" {
                n120 = Variant To Data(error in=w361, type=0.0 ("Magnet Return"), Variant=w363) -> (data=→"Instrument Response":dbl, error out=w357:errorcluster)
              }
            }
            n121 = call <vilib>:"Add State(s) to Queue__jki_lib_state_machine.vi"("State(s) in Front (\"\")"=w339, "State(s) in (\"\")"=w343) -> ("States Out"=w342:string)  [unwired: 13 in]
          }
        }
      }
    }
    frame Error {
    }
  }
  n122 = call-parent "Process.vi"("error in"=w8, "Instrument UI in"=w7) -> ("error out"=w5:errorcluster, "Instrument UI out"=→"Example Instrument UI out":refnum<class "LevyLab Instrument UI.lvclass">)  [unwired: 8 in]
  n123 = Merge Errors(w5, w4) -> (→"error out":errorcluster)
